vi "delay.vi"(7 "Delay Settings":T2 {"Wet/Dry" scale=0.0..5.0}, 9 "Audio R In":i16[](array[numeric]), 10 "Audio L In":i16[](array[numeric]), 11 "Effects":T1 {"Delay 2" scale=0.0..10.0; "Delay" scale=0.0..1.0}) -> (1 "Audio R Out":i16[](array[numeric]), 2 "Audio L Out":i16[](array[numeric]))   [LabVIEW 2014]
uses:
  Controls/Delay Controls.ctl
  Controls/Track Effects Settings.ctl
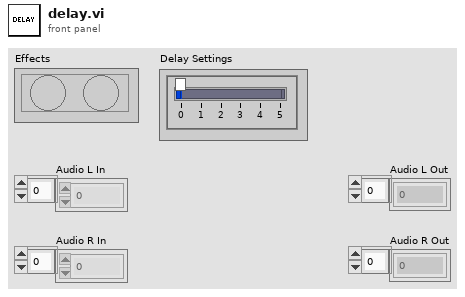
[diagram p1: front panel]
types:
  T1 = typedef "Track Effects Settings.ctl" = cluster{"Delay":dbl, "Delay 2":dbl}
  T2 = typedef "Delay Controls.ctl" = cluster{"Wet/Dry":u8}
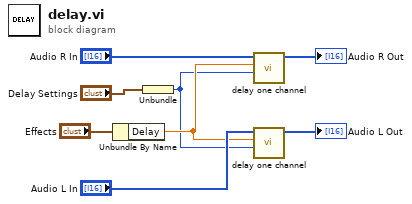
[diagram p0: block diagram]
diagram:
  n1 = Unbundle By Name("Effects") -> ("Delay"=w2:dbl)
  n2 = Unbundle("Delay Settings") -> ("Wet/Dry"=w1:u8)
  n3 = call "delay one channel.vi"("Delay"=w1, "Wet/Dry"=w2, "Audio In"="Audio R In") -> ("Audio Out"=→"Audio R Out":i16[])  [unwired: 8 in]
  n4 = call "delay one channel.vi"("Delay"=w1, "Wet/Dry"=w2, "Audio In"="Audio L In") -> ("Audio Out"=→"Audio L Out":i16[])  [unwired: 8 in]
